vi "Create User.vi"(8 "error in (no error)":errorcluster caption="错误输入（无错误）", 11 "Abstract Factory 输入":refnum<class "Abstract Factory.lvclass">) -> (0 "error out":errorcluster caption="错误输出", 2 "Abstract User.lvclass":refnum<class "Abstract User.lvclass">, 3 "Abstract Factory 输出":refnum<class "Abstract Factory.lvclass">)   [LabVIEW 2017, in "Abstract Factory.lvclass"]
uses:
  Abstract Factory.lvclass
  Abstract User/Abstract User.lvclass
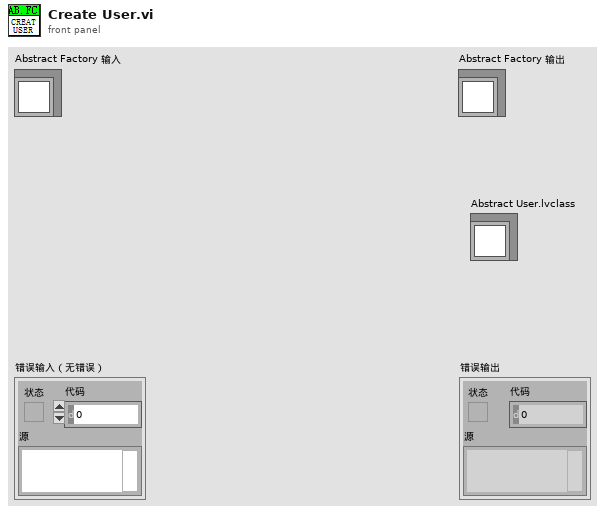
[diagram p1: front panel]
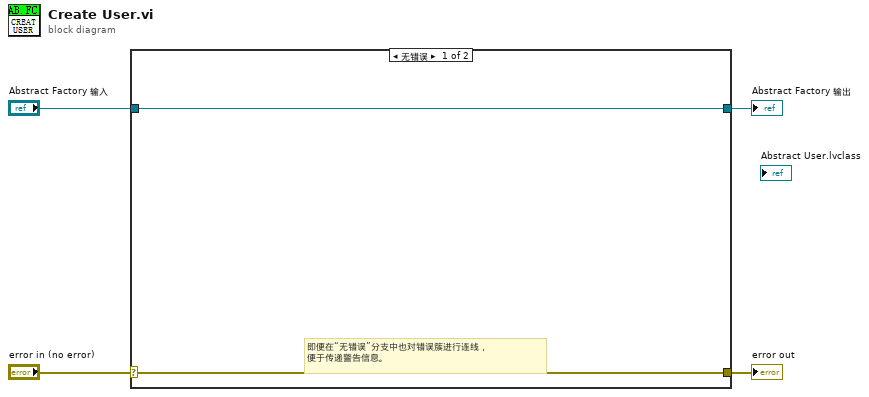
[diagram p0: block diagram]
diagram:
  n1 = case shown="无错误" "error in (no error)" {
    selector: "error in (no error)" -> [w6 w8]
    tunnel: [w6 w8] -> w3
    tunnel: [w5 w7] -> w1
    tunnel: "Abstract Factory 输入" -> [w5 w7]
    frame No Error {
      # "即便在“无错误”分支中也对错误簇进行连线，\n便于传递警告信息。"
    }
    frame Error {
    }
  }
  "error out" <- w3
  "Abstract Factory 输出" <- w1
